vi "Diagnostics.Restart.Loop.vi"(8 "error in (no error)":errorcluster, 11 "State Variables Out":T1={"Comm"=refnum, "Parameters"={"Properties"={"Name"="", "CAN"={"Interface"="", "Baud Rate"=0, "Diagnostic Protocol"=enum."GMLAN", "Transport Protocol"=enum."ISO TP - Normal Mode", "Transmit ID"=0, "Receive ID"=0, "Transmit Extension"=2, "Receive Extension"=1, "Receive UUDT ID"=0, "Enable Stream"=TRUE, "VW TP Channel ID"=0, "Fill Frame"=FALSE, "Fill Byte"=255, "Termination"=FALSE, "LIN Cluster"="ADCS_LIN_database", "NAD"=1, "IO Mode"=0, "Max DLC"=8, "FD Baud Rate"=0, "Security"={"Source DLL Path"=path "", "Security Level"=0, "Target DLL Path"=path ""}}, "986x"={"Enable"=FALSE, "RIO Device"="", "Bitfile"=path ""}, "Reads"=[], "Frames Lookup"=variant(enum16{"GMLAN", "KWP-2000", "UDS"} enum."GMLAN"), "Writes"=[], "DPIDs"=[], "DPID Lookup"=variant(u32 0), "DTC"={"Descriptor"={"DTC Byte Length"=2, "Status Byte Length"=1, "Add Data Byte Length"=1, "Byte Order"=enum."Motorola"}, "Value.Code"=[], "Value.String"=[], "Value.J2012String"=[], "Status.Code"=[], "Status.String"=[]}, "Created DTCs"=0}}, "ADCS Connection"={"Diag CAN Handle"=0, "Transport Protocol"=enum."ISO TP - Normal Mode", "Receive Address Extension"=0, "Transmit Address Extension"=0, "Receive CAN Id"=0, "Transmit CAN Id"=0, "Log Frames ?"=FALSE, "My TP Address"=0, "Other TP Address"=0, "T1"=0, "T2"=0, "T3"=0, "T4"=0, "Tx SN"=0, "Block Size"=0, "Rx SN"=0, "VW TP Initialized?"=FALSE, "Tx block no"=0, "baud rate"=0, "Interface"="", "Channel Diag CAN Handle"=0, "UDP Connection ID"=refnum, "TCP Connection ID"=refnum, "Target IP Addr"=0, "Source Address"=0, "Target Address"=0, "Send Header NACK?"=FALSE, "DLL Handle"=0, "NAD"=0, "Time Stamp read first"=0.0, "Time Stamp read last"=0.0, "Time Stamp write first"=0.0, "Time Stamp write last"=0.0, "Time Stamp write"=0.0, "Time Stamp read"=0.0, " I/O Mode"=0, "FD Baudrate"=0, "TX_DL"=8, "RX_DL"=8, "DoIP Protocol Version"=1, " Selected I/O Mode"=0, "TesterPresent Counter"=0, "TesterPresent Limit"=0, "TesterPresent Tick[ms]"=10, "TesterPresent RequireResponse?"=FALSE, "TesterPresent Stored Ref?"=FALSE, "TesterPresent Message"=[], "TesterPresent Task Handle"=0, "TesterPresent Semaphore"=refnum, "Response Plausibility Check"=1, "Default Version?"=TRUE, "Diagostic Globals"={"Timeout FC (Bs)"=250, "Timeout CF (Cr)"=250, "Timeout Diag Command"=1000, "Receive Block Size (BS)"=0, "Wait Time CF (STmin)"=5, "Max Waits (N_WFTmax)"=10, "Waits to Send (N_WAIT)"=0, "Time between Waits (TW)"=25, "Fill CAN Frames?"=TRUE, "Fill Byte"=255, "Invalid Response as Error?"=FALSE, "Max RspPending Count"=5, "VWTP Command Timeout"=50, "Transport Protocol"=enum."Diagnostics on IP", "Diag CAN Handle"=0, "DLL Handle"=0, "Timeout RspPending"=1000}, "Session-based Properties?"=FALSE}, "XNET References"={"Database"="", "GMLAN DPID Session"="", "Cluster"=""}, "XNETEngine (GMLAN)"=refnum, "Process"=refnum, "Reads"=refnum, "Writes"=refnum, "Cmds"=refnum, "DTCs"=refnum, "DTC Count"=refnum, "Status"=refnum, "Triggers"=refnum, "CANConnected"=refnum, "LocalStop"=refnum, "LocalCommStatus"=refnum} {"ADCS Connection"."Diagostic Globals"."Fill Byte" format="%x"; "ADCS Connection"."TesterPresent Message" format="%.0x"; "ADCS Connection"."Selected I/O Mode" items=["CAN", "CAN FD", "CAN FD+BRS", "ECU Determined"]; "ADCS Connection"."DoIP Protocol Version" items=["2010"=1, "2012"=2]; "ADCS Connection"."RX_DL" items=["8"=8, "12"=12, "16"=16, "20"=20, "24"=24, "32"=32, "48"=48, "64"=64]; "ADCS Connection"."TX_DL" items=["8"=8, "12"=12, "16"=16, "20"=20, "24"=24, "32"=32, "48"=48, "64"=64]; "ADCS Connection"."I/O Mode" items=["CAN", "CAN FD", "CAN FD+BRS", "Not yet determined"]; "Parameters"."Properties"."Writes"."Signals"."Byte Order" items=["Little Endian", "Big Endian"]; "Parameters"."Properties"."Writes"."Signals"."Data Type" items=["Signed", "Unsigned", "IEEE Float"]; "Parameters"."Properties"."CAN"."IO Mode" items=["CAN 2.0", "CAN FD", "CAN FD+BRS"]; "Parameters"."Properties"."CAN"."Fill Byte" format="%.0x"; "Parameters"."Properties"."CAN"."VW TP Channel ID" format="%.0x"; "Parameters"."Properties"."CAN"."Receive UUDT ID" format="%.0x"; "Parameters"."Properties"."CAN"."Receive Extension" format="%.0x"; "Parameters"."Properties"."CAN"."Transmit Extension" format="%.0x"; "Parameters"."Properties"."CAN"."Receive ID" format="%.0x"; "Parameters"."Properties"."CAN"."Transmit ID" format="%.0x"; "Parameters"."Properties"."Reads"."Signals"."Byte Order" items=["Little Endian", "Big Endian"]; "Parameters"."Properties"."Reads"."Signals"."Data Type" items=["Signed", "Unsigned", "IEEE Float"]}) -> (0 "Error Out":errorcluster)   [LabVIEW 2019, in "Diagnostics Addon Engine.lvlib"]
uses:
  Diagnostics Addon Engine.lvlib
  Types/Diagnostics.State.ctl
  <vilib>/NI/NIVS Addon Network Comm/Engine/VeriStand Comm.lvclass
  <vilib>/NI/NIVS Inline Async API/_VS Inline Async API/Process/Process.lvclass
  Shared/Types/SysDef.Compile.ctl
  Shared/Types/SysDef.Compile.Properties.ctl
  Shared/Types/CAN.ctl
  Shared/Types/CAN.Interface.ctl
  Shared/Types/Protocol.ctl
  Shared/Types/Transport.ctl
  Shared/Types/Security.ctl
  Shared/Types/986x.ctl
  Shared/Types/Frame.Compile.ctl
  Shared/Types/Type.ctl
  Shared/Types/Signal.ctl
  Shared/Types/DPID.ctl
  Shared/Types/DPID.Rate.ctl
  Shared/Types/DTC.Settings.ctl
  Shared/Types/DTC.Descriptor.ctl
  <vilib>/Automotive Diagnostic Command Set/Diagnostic Transport.llb/Diag Reference.ctl
  <vilib>/Automotive Diagnostic Command Set/Diagnostic Transport.llb/Transport Protocol Selector.ctl
  <vilib>/Automotive Diagnostic Command Set/Diagnostic Transport.llb/DoIP Protocol Version.ctl
  <vilib>/Automotive Diagnostic Command Set/Diagnostic Transport.llb/Diag Globals.ctl
  Types/XNET.Refs.ctl
  <vilib>/NI/AMC/Message Queue.ctl
  <vilib>/NI/AMC/Message.ctl
  <vilib>/NI/Tools/Keyed Array/KeyedArray.ctl
  <vilib>/NI/NIVS Inline Async API/_Data Access Engine/Data Access Engine/Types/Write.DVR.ctl
  <vilib>/NI/NIVS Inline Async API/_Data Access Engine/Access Type Classes/Write/Write.lvclass
  <vilib>/NI/NIVS Inline Async API/_Data Access Engine/Data Access Engine/Types/Read.DVR.ctl
  <vilib>/NI/NIVS Inline Async API/_Data Access Engine/Access Type Classes/Read/Read.lvclass
  <vilib>/NI/NIVS Inline Async API/_Data Access Engine/Data Access Engine/Types/ReadWrite.DVR.ctl
  <vilib>/NI/NIVS Inline Async API/_Data Access Engine/Access Type Classes/ReadWrite/ReadWrite.lvclass
  <vilib>/NI/NIVS Inline Async API/_Data Access Engine/Access Type Classes/Write/Write.lvclass/Write.ctl
  <vilib>/NI/NIVS Addon Network Comm/Engine/VeriStand Comm.lvclass/VeriStand Comm.ctl
  <vilib>/NI/NIVS Inline Async API/_VS Inline Async API/Process/Process.lvclass/Process.ctl
  <vilib>/NI/NIVS Inline Async API/_Data Access Engine/Access Type Classes/Read/Read.lvclass/Read.ctl
  <vilib>/NI/NIVS Inline Async API/_Data Access Engine/Data Access Engine/Methods/Write.Data.vi
  Diagnostics.Main.UUDT.Engine.vi
  Diagnostics.Main.CmdResp.Engine.vi
  <vilib>/NI/NIVS Inline Async API/_VS Inline Async API/Error Handling Process/SubVIs/Error.ConvertArray.vi
  <vilib>/NI/NIVS Inline Async API/_Data Access Engine/Access Type Classes/Write/Write.ProcessData.vi
  <vilib>/NI/AMC/Read Next Message.vi
  <vilib>/NI/Tools/Keyed Array/Index.vi
  Frames.Refs.Cleanup.vi
  Status.Set.vi
  Signals.Scale.EU.vi
  <vilib>/NI/NIVS Inline Async API/_Data Access Engine/Data Access Engine/Methods/Write.Data.Commit.vi
  GMLAN/Utilities/Convert Data to DTCs.vi
  <vilib>/NI/NIVS Addon Network Comm/Engine/Comm API/Send Command.vi
  DTCs.List.Update.vi
  Restart.LocalStop.Read.vi
  GMLAN/_SubVIs/ReadDiagnosticInformation_ByStatus.vi
  GMLAN/_SubVIs/ReadDiagnosticInformation_sendOnChangeDTCCount.vi
  GMLAN/_SubVIs/ReadFailureRecordData_readFailureRecordParameters.vi
  GMLAN/_SubVIs/ReadDiagnosticInformation_readStatusOfDTCByDTCNumber.vi
  GMLAN/GMLAN DynamicallyDefineMessage.vi
  GMLAN/GMLAN ReadDataByPacketIdentifier.vi
  GMLAN/GMLAN ReadDataByParameterIdentifier.vi
  <vilib>/NI/AMC/Send Local Message.vi
  Signals.Scale.Raw.vi
  GMLAN/GMLAN DeviceControl.vi
  GMLAN/GMLAN TesterPresent.vi
  GMLAN/GMLAN InitiateDiagnosticOperation.vi
  GMLAN/GMLAN DisableNormalCommunication.vi
  GMLAN/GMLAN ReturnToNormalMode.vi
  ADCS.UnlockECUSecurity.vi
  <vilib>/NI/NIVS Addon Network Comm/Engine/Comm API/Respond to Command.vi
  DTC.Descriptor.Override.vi
  GMLAN/GMLAN ClearDiagnosticInformation.vi
  GMLAN/GMLAN ReadDataByIdentifier.vi
  Frames.Lookup.Size.Get.vi
  ADCS.TesterPresent.vi
  <vilib>/NI/AMC/Read Termination Message.vi
  <vilib>/NI/Tools/Keyed Array/Map String.vi
  ADCS.Get.ErrorByte.vi
  <vilib>/NI/NIVS Inline Async API/_Data Access Engine/Data Access Engine/Methods/Write.Data.Buffer.vi
  <vilib>/NI/NIVS Inline Async API/_Data Access Engine/Access Type Classes/Write/Write.Commit.vi
  GMLAN/Utilities/Convert Raw Data to DTCs.vi
  <vilib>/Utility/error.llb/Clear Errors.vi
  <vilib>/NI/AMC/Create Single Message.vi
  <vilib>/NI/AMC/Update Message Routing Info.vi
  <vilib>/NI/NIVS Inline Async API/_Data Access Engine/Data Access Engine/Methods/Read.Data.vi
  GMLAN/Utilities/GMLAN Service Broadcast.vi
  Security.DLL.vi
  GMLAN/GMLAN SecurityAccess.vi
  GMLAN/_SubVIs/SecurityAccess_sendKey.vi
  GMLAN/_SubVIs/SecurityAccess_requestSeed.vi
  <vilib>/NI/Tools/String/Get Case Matching.vi
  <vilib>/NI/NIVS Inline Async API/_Data Access Engine/Access Type Classes/Write/Write.Buffer.vi
  <vilib>/NI/NIVS Inline Async API/_Data Access Engine/Access Type Classes/Read/Read.ProcessData.vi
  <vilib>/Automotive Diagnostic Command Set/Diagnostic Transport.llb/Diagnostic Service Send.vi
  <vilib>/Automotive Diagnostic Command Set/Diagnostic Transport.llb/Diagnostic Response Recv.vi
  <vilib>/Automotive Diagnostic Command Set/Diagnostic Transport.llb/ISOTP Transmit.vi
  <vilib>/Automotive Diagnostic Command Set/Diagnostic Transport.llb/ISOTP7 Transmit.vi
  <vilib>/Automotive Diagnostic Command Set/Diagnostic Transport.llb/DoIP Transmit.vi
  <vilib>/Automotive Diagnostic Command Set/Diagnostic Transport.llb/LIN ISOTP Transmit.vi
  <vilib>/Automotive Diagnostic Command Set/Diagnostic Transport.llb/Diagnostic Service Recv.vi
  <vilib>/Automotive Diagnostic Command Set/Diagnostic Transport.llb/ISOTP Send FF.vi
  <vilib>/Automotive Diagnostic Command Set/Diagnostic Transport.llb/ISOTP Send CFs.vi
  <vilib>/Automotive Diagnostic Command Set/Diagnostic Transport.llb/ISOTP Send Frame.vi
  <vilib>/Automotive Diagnostic Command Set/Diagnostic Transport.llb/ISOTP7 Send FF.vi
  <vilib>/Automotive Diagnostic Command Set/Diagnostic Transport.llb/ISOTP7 Send CFs.vi
  <vilib>/Automotive Diagnostic Command Set/Diagnostic Transport.llb/ISOTP7 Send Frame.vi
  <vilib>/Automotive Diagnostic Command Set/Diagnostic Transport.llb/DoIP TCP Msg Send.vi
  <vilib>/Automotive Diagnostic Command Set/Diagnostic Transport.llb/DoIP TCP Msg Recv.vi
  <vilib>/Automotive Diagnostic Command Set/Diagnostic Transport.llb/DoIP Check Addresses.vi
  <vilib>/Automotive Diagnostic Command Set/Diagnostic Transport.llb/DoIP Check ACK Code.vi
  <vilib>/Automotive Diagnostic Command Set/Diagnostic Transport.llb/ISOTP Receive.vi
  <vilib>/Automotive Diagnostic Command Set/Diagnostic Transport.llb/ISOTP7 Receive.vi
  <vilib>/Automotive Diagnostic Command Set/Diagnostic Transport.llb/DoIP Receive.vi
  <vilib>/Automotive Diagnostic Command Set/Diagnostic Transport.llb/LIN ISOTP Receive.vi
  <vilib>/Automotive Diagnostic Command Set/Diagnostic Transport.llb/Diag Get Globals.vi
  <vilib>/Automotive Diagnostic Command Set/Diagnostic Transport.llb/ISOTP Recv FC.vi
  <vilib>/Automotive Diagnostic Command Set/Diagnostic Transport.llb/ISOTP Send CF.vi
  <vilib>/Automotive Diagnostic Command Set/Diagnostic Transport.llb/Diag Fill Frame.vi
  <vilib>/Automotive Diagnostic Command Set/Diagnostic Transport.llb/ISOTP Calc Send Params.vi
  <vilib>/Automotive Diagnostic Command Set/Diagnostic Transport.llb/ISOTP7 Recv FC.vi
  <vilib>/Automotive Diagnostic Command Set/Diagnostic Transport.llb/ISOTP7 Send CF.vi
  <vilib>/Automotive Diagnostic Command Set/Diagnostic Transport.llb/DoIP Add Addresses.vi
  <vilib>/Automotive Diagnostic Command Set/Diagnostic Transport.llb/DoIP TCP Send.vi
  <vilib>/Automotive Diagnostic Command Set/Diagnostic Transport.llb/DoIP TCP Recv.vi
  <vilib>/Automotive Diagnostic Command Set/Diagnostic Transport.llb/DoIP Add Header.vi
  <vilib>/Automotive Diagnostic Command Set/Diagnostic Transport.llb/ISOTP Recv Frame.vi
  <vilib>/Automotive Diagnostic Command Set/Diagnostic Transport.llb/ISOTP Recv CFs.vi
  <vilib>/Automotive Diagnostic Command Set/Diagnostic Transport.llb/ISOTP7 Recv Frame.vi
  <vilib>/Automotive Diagnostic Command Set/Diagnostic Transport.llb/ISOTP7 Recv CFs.vi
  <vilib>/Automotive Diagnostic Command Set/Diagnostic Transport.llb/DoIP Send Alive.vi
  <vilib>/Automotive Diagnostic Command Set/Diagnostic Transport.llb/DoIP Check Error.vi
  <vilib>/Automotive Diagnostic Command Set/Diagnostic Transport.llb/ISOTP Check Redo.vi
  <vilib>/Automotive Diagnostic Command Set/Diagnostic Transport.llb/ISOTP Recv Block.vi
  <vilib>/Automotive Diagnostic Command Set/Diagnostic Transport.llb/ISOTP7 Recv Block.vi
  <vilib>/Automotive Diagnostic Command Set/Diagnostic Transport.llb/ISOTP Send FC.vi
  <vilib>/Automotive Diagnostic Command Set/Diagnostic Transport.llb/ISOTP Add CF.vi
  <vilib>/Automotive Diagnostic Command Set/Diagnostic Transport.llb/ISOTP7 Send FC.vi
  <vilib>/Automotive Diagnostic Command Set/Diagnostic Transport.llb/ISOTP7 Add CF.vi
  <vilib>/NI/NIVS Addon Network Comm/Shared/Comm Constants.vi
  <vilib>/NI/AMC/Globals.vi
  <vilib>/Automotive Diagnostic Command Set/Diagnostic Transport.llb/Diag Get Property.vi
  <vilib>/Automotive Diagnostic Command Set/Diagnostic Transport.llb/Diag Set Property.vi
  <vilib>/Automotive Diagnostic Command Set/Diagnostic Transport.llb/Diagnostic Service.vi
  <vilib>/Automotive Diagnostic Command Set/Diagnostic Transport.llb/Apply Success Failure Error.vi
  DPIDs.IDs.Sort.vi
  <vilib>/NI/AMC/Send Message.vi
  Shared/SubVIs/Constants.vi
  <vilib>/xnet/xnet.llb/XNET Convert.vi
  <vilib>/xnet/xnet.llb/XNET Convert (Signal to Frame CAN).vi
  <vilib>/Automotive Diagnostic Command Set/Diagnostic Protocols.llb/TesterPresent.vi
  <vilib>/Automotive Diagnostic Command Set/Diagnostic Transport.llb/Diag Globals.vi
  <vilib>/Automotive Diagnostic Command Set/Diagnostic Transport.llb/CAN Send Frame Check Queue.vi
  <vilib>/Automotive Diagnostic Command Set/Diagnostic Transport.llb/Diag CAN get timestamp.vi
  <vilib>/Automotive Diagnostic Command Set/Diagnostic Transport.llb/Diag CAN read.vi
  <vilib>/Automotive Diagnostic Command Set/Diagnostic Transport.llb/ISOTP Calc Actual IO Mode.vi
  <vilib>/Automotive Diagnostic Command Set/Diagnostic Transport.llb/ISOTP Get FC Data.vi
  <vilib>/Automotive Diagnostic Command Set/Diagnostic Transport.llb/VWTP Write.vi
  <vilib>/Automotive Diagnostic Command Set/Diagnostic Transport.llb/DoIP Analyze Header.vi
  <vilib>/Automotive Diagnostic Command Set/Diagnostic Transport.llb/Diag CAN status.vi
  <vilib>/Automotive Diagnostic Command Set/Diagnostic Transport.llb/VWTP Read.vi
  <vilib>/Automotive Diagnostic Command Set/Diagnostic Transport.llb/Apply Diagnostic Error.vi
  <vilib>/Automotive Diagnostic Command Set/Diagnostic Protocols.llb/UDS TesterPresent.vi
  <vilib>/Automotive Diagnostic Command Set/Diagnostic Protocols.llb/UDS DiagnosticSessionControl.vi
  <vilib>/Automotive Diagnostic Command Set/Diagnostic Protocols.llb/StartDiagnosticSession.vi
  <vilib>/Automotive Diagnostic Command Set/Diagnostic Protocols.llb/StopDiagnosticSession.vi
  <vilib>/Automotive Diagnostic Command Set/Diagnostic Protocols.llb/UDS CommunicationControl.vi
  <vilib>/Automotive Diagnostic Command Set/Diagnostic Protocols.llb/DisableNormalMessageTransmission.vi
  <vilib>/Automotive Diagnostic Command Set/Diagnostic Protocols.llb/EnableNormalMessageTransmission.vi
  <vilib>/Automotive Diagnostic Command Set/Diagnostic Protocols.llb/UDS RequestSeed.vi
  <vilib>/Automotive Diagnostic Command Set/Diagnostic Protocols.llb/RequestSeed.vi
  <vilib>/Automotive Diagnostic Command Set/Diagnostic Protocols.llb/UDS SendKey.vi
  <vilib>/Automotive Diagnostic Command Set/Diagnostic Protocols.llb/SendKey.vi
  <vilib>/Automotive Diagnostic Command Set/Diagnostic Protocols.llb/UDS ReportDTCBySeverityMaskRecord.vi
  <vilib>/Automotive Diagnostic Command Set/Diagnostic Protocols.llb/UDS ReportSeverityInformationOfDTC.vi
  <vilib>/Automotive Diagnostic Command Set/Diagnostic Protocols.llb/UDS ReportDTCByStatusMask.vi
  <vilib>/Automotive Diagnostic Command Set/Diagnostic Protocols.llb/ReadStatusOfDTC.vi
  <vilib>/Automotive Diagnostic Command Set/Diagnostic Protocols.llb/ReadDTCByStatus.vi
  <vilib>/Automotive Diagnostic Command Set/Diagnostic Protocols.llb/ClearDiagnosticInformation.vi
  <vilib>/Automotive Diagnostic Command Set/Diagnostic Protocols.llb/UDS ClearDiagnosticInformation.vi
  <vilib>/Automotive Diagnostic Command Set/Diagnostic Protocols.llb/ReadDataByLocalIdentifier.vi
  <vilib>/Automotive Diagnostic Command Set/Diagnostic Protocols.llb/UDS ReadDataByIdentifier.vi
  <vilib>/xnet/xnet.llb/XNET Convert (Frame CAN to Signal).vi
  <vilib>/Automotive Diagnostic Command Set/Diagnostic Protocols.llb/WriteDataByLocalIdentifier.vi
  <vilib>/Automotive Diagnostic Command Set/Diagnostic Protocols.llb/UDS WriteDataByIdentifier.vi
  <vilib>/Automotive Diagnostic Command Set/Diagnostic Protocols.llb/UDS ControlDTCSetting.vi
  <vilib>/Automotive Diagnostic Command Set/Diagnostic Protocols.llb/ControlDTCSetting.vi
  <vilib>/Automotive Diagnostic Command Set/Diagnostic Protocols.llb/ECUReset.vi
  <vilib>/Automotive Diagnostic Command Set/Diagnostic Protocols.llb/UDS ECUReset.vi
  <vilib>/Automotive Diagnostic Command Set/Diagnostic Protocols.llb/ReadMemoryByAddress.vi
  <vilib>/Automotive Diagnostic Command Set/Diagnostic Protocols.llb/UDS06 ReadMemoryByAddress.vi
  <vilib>/Automotive Diagnostic Command Set/Diagnostic Protocols.llb/UDS ReadMemoryByAddress.vi
  <vilib>/Automotive Diagnostic Command Set/Diagnostic Protocols.llb/WriteMemoryByAddress.vi
  <vilib>/Automotive Diagnostic Command Set/Diagnostic Protocols.llb/UDS06 WriteMemoryByAddress.vi
  <vilib>/Automotive Diagnostic Command Set/Diagnostic Protocols.llb/UDS WriteMemoryByAddress.vi
  <vilib>/Automotive Diagnostic Command Set/Diagnostic Protocols.llb/InputOutputControlByLocalIdentifier.vi
  <vilib>/Automotive Diagnostic Command Set/Diagnostic Protocols.llb/UDS InputOutputControlByIdentifier.vi
  <vilib>/Automotive Diagnostic Command Set/Diagnostic Protocols.llb/StartRoutineByLocalIdentifier.vi
  <vilib>/Automotive Diagnostic Command Set/Diagnostic Protocols.llb/UDS RoutineControl.vi
  <vilib>/Automotive Diagnostic Command Set/Diagnostic Protocols.llb/RequestRoutineResultsByLocalIdentifier.vi
  <vilib>/Automotive Diagnostic Command Set/Diagnostic Protocols.llb/StopRoutineByLocalIdentifier.vi
  <vilib>/xnet/xnet.llb/XNET Read.vi
  <vilib>/xnet/xnet.llb/XNET Read (Frame CAN).vi
  <vilib>/Automotive Diagnostic Command Set/Diagnostic Protocols.llb/Convert to Phys.vi
  <vilib>/xnet/xnet.llb/XNET Clear.vi
  <vilib>/xnet/xnet.llb/XNET Database Delete Object.vi
  <vilib>/xnet/xnet.llb/XNET Database Delete (Cluster).vi
  <vilib>/xnet/xnet.llb/XNET Database Close.vi
  <vilib>/xnet/xnet.llb/XNET Database Close (Database).vi
  <vilib>/Automotive Diagnostic Command Set/Diagnostic Transport.llb/Close Diagnostic.vi
  <vilib>/NI VeriStand/Custom Device Tools/Custom Device Utility Library/Custom Device Utility Library.lvlib
  <vilib>/NI/NIVS Inline Async API/_Data Access Engine/Data Access Engine/Data Access Engine.lvclass
  Shared/Diagnostics Addon Shared.lvlib
  <vilib>/addons/Automotive Diagnostic Command Set/NI_Automotive Diagnostic Command Set.lvlib
  <vilib>/NI/Tools/Keyed Array/Tools_KeyedArray.lvlib
  <vilib>/NI/AMC/AMC.lvlib
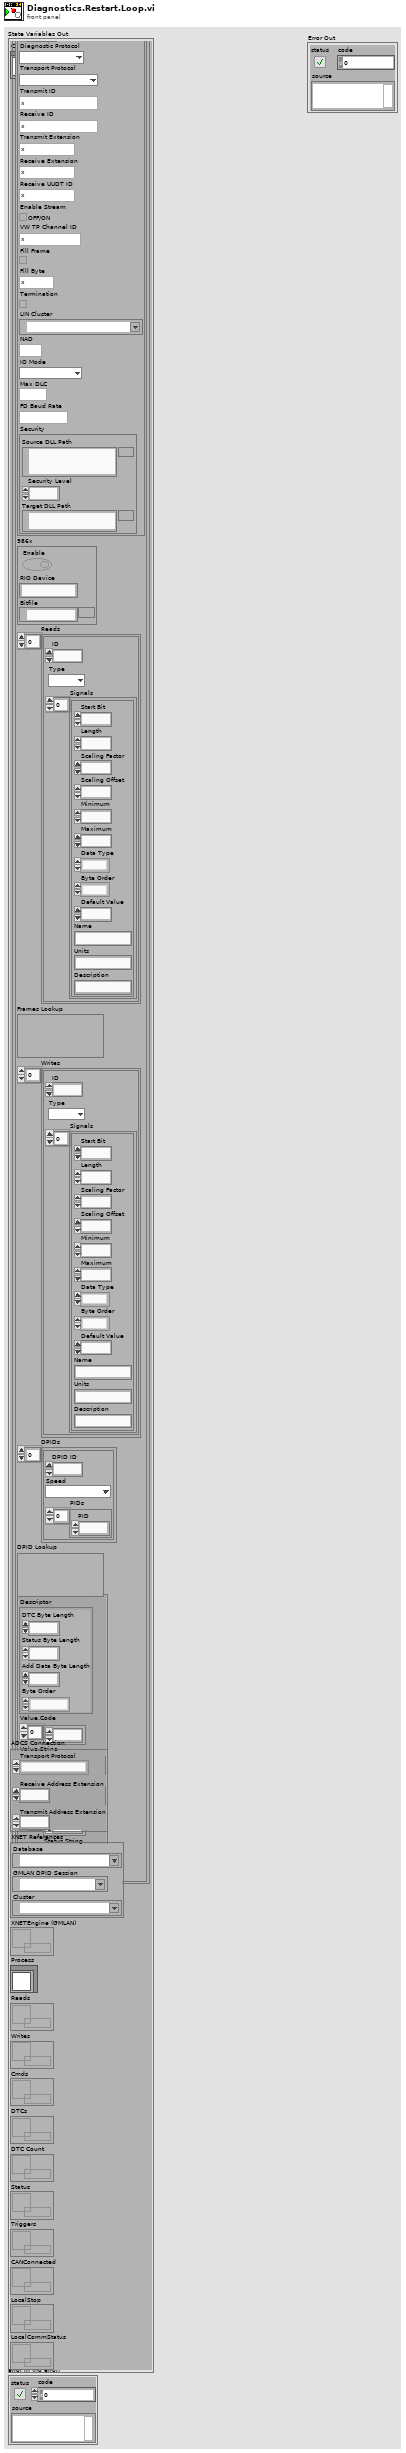
[diagram p1: front panel]
types:
  T1 = typedef "Diagnostics Addon Engine.lvlib/Diagnostics.State.ctl" = cluster{"Comm":refnum<class "VeriStand Comm.lvclass">, "Parameters":T2, "ADCS Connection":T17, "XNET References":T22, "XNETEngine (GMLAN)":T23, "Process":refnum<class "Process.lvclass">, "Reads":T24, "Writes":T25, "Cmds":T26, "DTCs":T24, "DTC Count":T24, "Status":T24, "Triggers":T26, "CANConnected":T24, "LocalStop":refnum<data-value>, "LocalCommStatus":refnum<data-value>}
  T2 = typedef "Diagnostics Addon Shared.lvlib/SysDef.Compile.ctl" = cluster{"Properties":T3}
  T3 = typedef "Diagnostics Addon Shared.lvlib/SysDef.Compile.Properties.ctl" = cluster{"Name":string, "CAN":T4, "986x":T9, "Reads":T10[], "Frames Lookup":variant, "Writes":T10[], "DPIDs":T13[], "DPID Lookup":variant, "DTC":T15, "Created DTCs":u32}
  T4 = typedef "Diagnostics Addon Shared.lvlib/CAN.ctl" = cluster{"Interface":T5, "Baud Rate":u64, "Diagnostic Protocol":T6, "Transport Protocol":T7, "Transmit ID":u32, "Receive ID":u32, "Transmit Extension":u8, "Receive Extension":u8, "Receive UUDT ID":u32, "Enable Stream":bool, "VW TP Channel ID":u32, "Fill Frame":bool, "Fill Byte":u8, "Termination":bool, "LIN Cluster":refnum<k21>, "NAD":u8, "IO Mode":u32, "Max DLC":u16, "FD Baud Rate":u64, "Security":T8}
  T5 = typedef "Diagnostics Addon Shared.lvlib/CAN.Interface.ctl" = string
  T6 = typedef "Diagnostics Addon Shared.lvlib/Protocol.ctl" = enum16{"GMLAN", "KWP-2000", "UDS", "User-Defined"}
  T7 = typedef "Diagnostics Addon Shared.lvlib/Transport.ctl" = enum16{"ISO TP - Normal Mode", "ISO TP - Mixed Mode", "VW TP 2.0", "Diagnostics on IP", "ISO TP LIN"}
  T8 = typedef "Diagnostics Addon Shared.lvlib/Security.ctl" = cluster{"Source DLL Path":path, "Security Level":u8, "Target DLL Path":path}
  T9 = typedef "Diagnostics Addon Shared.lvlib/986x.ctl" = cluster{"Enable":bool, "RIO Device":string, "Bitfile":path}
  T10 = typedef "Diagnostics Addon Shared.lvlib/Frame.Compile.ctl" = cluster{"ID":u32, "Type":T11, "Signals":T12[]}
  T11 = typedef "Diagnostics Addon Shared.lvlib/Type.ctl" = enum16{"DID", "CDID", "PID", "CPID", "Read Memory", "Write Memory", "DTC Control", "IO Cmd", "IO Resp", "Routine Start Cmd", "Routine Start Resp", "Routine Request Cmd", "Routine Request Resp", "Routine Stop Cmd", "Routine Stop Resp", "UserDefined Cmd", "UserDefined Rsp"}
  T12 = typedef "Diagnostics Addon Shared.lvlib/Signal.ctl" = cluster{"Start Bit":u32, "Length":u32, "Scaling Factor":dbl, "Scaling Offset":dbl, "Minimum":dbl, "Maximum":dbl, "Data Type":u32, "Byte Order":u32, "Default Value":dbl, "Name":string, "Units":string, "Description":string}
  T13 = typedef "Diagnostics Addon Shared.lvlib/DPID.ctl" = cluster{"DPID ID":u8, "Speed":T14, "PIDs":u16[]}
  T14 = typedef "Diagnostics Addon Shared.lvlib/DPID.Rate.ctl" = enum16{"Slow", "Medium", "Fast"}
  T15 = typedef "Diagnostics Addon Shared.lvlib/DTC.Settings.ctl" = cluster{"Descriptor":T16, "Value.Code":dbl[], "Value.String":string[], "Value.J2012String":string[], "Status.Code":dbl[], "Status.String":string[]}
  T16 = typedef "Diagnostics Addon Shared.lvlib/DTC.Descriptor.ctl" = cluster{"DTC Byte Length":i32, "Status Byte Length":i32, "Add Data Byte Length":i32, "Byte Order":enum16{"Motorola", "Intel"}}
  T17 = typedef "NI_Automotive Diagnostic Command Set.lvlib/Diag Reference.ctl" = cluster{"Diag CAN Handle":u32, "Transport Protocol":T18, "Receive Address Extension":u8, "Transmit Address Extension":u8, "Receive CAN Id":u32, "Transmit CAN Id":u32, "Log Frames ?":bool, "My TP Address":u8, "Other TP Address":u8, "T1":u16, "T2":u16, "T3":u16, "T4":u16, "Tx SN":u8, "Block Size":u8, "Rx SN":u8, "VW TP Initialized?":bool, "Tx block no":u8, "baud rate":u64, "Interface":string, "Channel Diag CAN Handle":u32, "UDP Connection ID":refnum<k16>, "TCP Connection ID":refnum<k5>, "Target IP Addr":u32, "Source Address":u16, "Target Address":u16, "Send Header NACK?":bool, "DLL Handle":u32, "NAD":u8, "Time Stamp read first":dbl, "Time Stamp read last":dbl, "Time Stamp write first":dbl, "Time Stamp write last":dbl, "Time Stamp write":dbl, "Time Stamp read":dbl, " I/O Mode":u32, "FD Baudrate":u64, "TX_DL":u16, "RX_DL":u16, "DoIP Protocol Version":T19, " Selected I/O Mode":u32, "TesterPresent Counter":u32, "TesterPresent Limit":u32, "TesterPresent Tick[ms]":i32, "TesterPresent RequireResponse?":bool, "TesterPresent Stored Ref?":bool, "TesterPresent Message":u8[], "TesterPresent Task Handle":i32, "TesterPresent Semaphore":T20, "Response Plausibility Check":u32, "Default Version?":bool, "Diagostic Globals":T21, "Session-based Properties?":bool}
  T18 = typedef "NI_Automotive Diagnostic Command Set.lvlib/Transport Protocol Selector.ctl" = enum16{"ISO TP - Normal Mode", "ISO TP - Mixed Mode", "VW TP 2.0", "Diagnostics on IP", "ISO TP LIN"}
  T19 = typedef "NI_Automotive Diagnostic Command Set.lvlib/DoIP Protocol Version.ctl" = u8
  T20 = typedef "Semaphore RefNum" = refnum<k1>
  T21 = typedef "NI_Automotive Diagnostic Command Set.lvlib/Diag Globals.ctl" = cluster{"Timeout FC (Bs)":u32, "Timeout CF (Cr)":u32, "Timeout Diag Command":u32, "Receive Block Size (BS)":u8, "Wait Time CF (STmin)":u8, "Max Waits (N_WFTmax)":u8, "Waits to Send (N_WAIT)":i32, "Time between Waits (TW)":u32, "Fill CAN Frames?":bool, "Fill Byte":u32, "Invalid Response as Error?":bool, "Max RspPending Count":u32, "VWTP Command Timeout":u32, "Transport Protocol":T18, "Diag CAN Handle":u32, "DLL Handle":u32, "Timeout RspPending":u32}
  T22 = typedef "Diagnostics Addon Engine.lvlib/XNET.Refs.ctl" = cluster{"Database":refnum<k21>, "GMLAN DPID Session":refnum<k21>, "Cluster":refnum<k21>}
  T23 = typedef "AMC.lvlib/Message Queue.ctl" = refnum<queue>
  T24 = typedef "Data Access Engine.lvlib/Data Access Engine.lvclass/Write.DVR.ctl" = refnum<data-value>
  T25 = typedef "Data Access Engine.lvlib/Data Access Engine.lvclass/Read.DVR.ctl" = refnum<data-value>
  T26 = typedef "Data Access Engine.lvlib/Data Access Engine.lvclass/ReadWrite.DVR.ctl" = refnum<data-value>
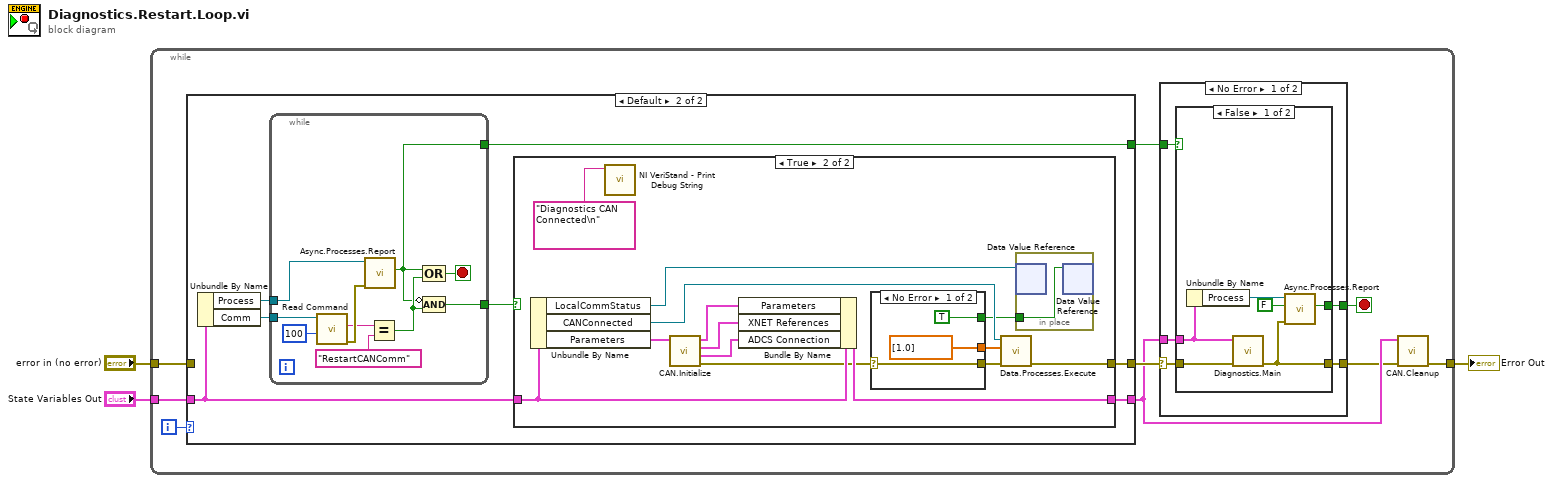
[diagram p0: block diagram]
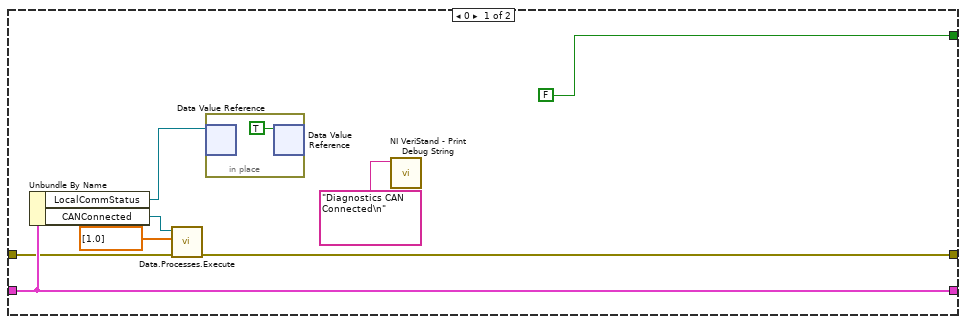
[diagram p2: hidden frame]
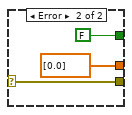
[diagram p4: hidden frame]
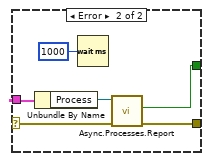
[diagram p6: hidden frame]
diagram:
  n1 = while {
    tunnel: "error in (no error)" -> [w12]
    tunnel: "State Variables Out" -> [w11]
    tunnel: [w5] -> w1
    i -> [w8]
    stop <- w9 stop-if-true
    n2 = case shown="Default" w8 {
      tunnel: [w20 w28] -> w7
      tunnel: w12 -> [w18 _]
      tunnel: w11 -> [w20 w26]
      tunnel: [w17 w27] -> w10
      tunnel: [FALSE w22] -> w4
      frame 0 {
        n3 = Unbundle By Name(w20) -> ("LocalCommStatus"=w13:refnum<data-value>, "CANConnected"=w19:T24)
        n4 = call-poly <vilib>:"Data.Processes.Execute.vi"("error in (no error)"=w18, "Values"=dbl[] [1.0], "Ref"=w19) -> ("error out"=w17:errorcluster)  [unwired: 8 in]
        n5 = in-place {
          n6 = in-place-dvr #1(w13) -> ()  [unwired: 2 out]
          n7 = in-place-dvr #1(TRUE ("data value")) -> ()  [unwired: 2 out]
        }
        n8 = call <vilib>:"NI VeriStand - Print Debug String.vi"("Message"="Diagnostics CAN Connected\n") -> ()  [unwired: 10 in, 1 out]
      }
      frame Default {
        n9 = Unbundle By Name(w26) -> ("Process"=w24:refnum<class "Process.lvclass">, "Comm"=w25:refnum<class "VeriStand Comm.lvclass">)
        n10 = while {
          tunnel: w25 -> [w59]
          tunnel: w24 -> [w58]
          tunnel: [w52] -> w23
          tunnel: [w51] -> w22
          stop <- w54 stop-if-true
          n11 = call <vilib>:"Read Command.vi"("timeout (100 ms)"=100 ("timeout (1ms)"), "VeriStand Comm in"=w59) -> ("error out"=w57:errorcluster, "message name"=w55:string)  [unwired: 4 in, 4 out]
          n12 = call <vilib>:"Async.Processes.Report.vi"("Error"=w57, "Process in"=w58) -> ("Stop"=w51:bool)  [unwired: 8 in, 1 out]
          n13 = Equal?(x=w55, y="RestartCANComm" ("Name")) -> (x = y?=w53:bool)
          n14 = Compound Arithmetic op=OR(w51, w53) -> (w54:bool)
          n15 = Compound Arithmetic op=AND(invert w51, w53) -> (w52:bool)
        }
        n16 = case shown="True" w23 {
          tunnel: [w29 w43] -> w28
          tunnel: [_ w37] -> w27
          tunnel: w26 -> [w29 w35]
          frame False {
          }
          frame True {
            n17 = Unbundle By Name(w35) -> ("LocalCommStatus"=w33:refnum<data-value>, "CANConnected"=w36:T24, "Parameters"=w42:T2)
            n18 = call <vilib>:"NI VeriStand - Print Debug String.vi"("Message"="Diagnostics CAN Connected\n") -> ()  [unwired: 10 in, 1 out]
            n19 = call "CAN.Initialize.vi"("Parameters"=w42) -> ("error out"=w32:errorcluster, "ADCS Connection"=w39:T17, "XNET References"=w40:T22, "Parameters"=w41:T2)  [unwired: 7 in]
            n20 = Bundle By Name(cluster=w35, "Parameters"=w41, "XNET References"=w40, "ADCS Connection"=w39) -> (w43:T1)
            n21 = case shown="No Error" w32 {
              selector: w32 -> [w45 w49]
              tunnel: [dbl[] [1.0] ("Values") dbl[] [0.0] ("Values")] -> w38
              tunnel: [w45 w49] -> w31
              tunnel: [TRUE FALSE] -> w30
              frame No Error {
              }
              frame Error {
              }
            }
            n22 = call-poly <vilib>:"Data.Processes.Execute.vi"("error in (no error)"=w31, "Values"=w38, "Ref"=w36) -> ("error out"=w37:errorcluster)  [unwired: 8 in]
            n23 = in-place {
              in-place-border: w30 -> [w50]
              n24 = in-place-dvr #2(w33) -> ()  [unwired: 2 out]
              n25 = in-place-dvr #2(w50) -> ()  [unwired: 2 out]
            }
          }
        }
      }
    }
    n26 = case shown="No Error" w10 {
      selector: w10 -> [w63 w75]
      tunnel: w7 -> [w65 w78]
      tunnel: [w64 w74] -> w9
      tunnel: [w62 w75] -> w6
      tunnel: w4 -> [w61 _]
      frame No Error {
        n27 = case shown="False" w61 {
          selector: w61 -> [_ w72]
          tunnel: w65 -> [w71 _]
          tunnel: [w70 w72] -> w64
          tunnel: w63 -> [w69 w73]
          tunnel: [w68 w73] -> w62
          frame False {
            n28 = Unbundle By Name(w71) -> ("Process"=w67:refnum<class "Process.lvclass">)
            n29 = call "Diagnostics.Main.vi"("error in (no error)"=w69, "State Variables"=w71) -> ("error out"=w68:errorcluster)  [unwired: 9 in]
            n30 = call <vilib>:"Async.Processes.Report.vi"("Error"=w68, "Stop Async on Error?"=FALSE ("Stop on Error?"), "Process in"=w67) -> ("Stop"=w70:bool)  [unwired: 7 in, 1 out]
          }
          frame True {
          }
        }
      }
      frame Error {
        n31 = Unbundle By Name(w78) -> ("Process"=w77:refnum<class "Process.lvclass">)
        n32 = Wait (ms)(milliseconds to wait=u32 1000 ("millisecond multiple")) -> ()  [unwired: 1 out]
        n33 = call <vilib>:"Async.Processes.Report.vi"("Error"=w75, "Process in"=w77) -> ("Stop"=w74:bool)  [unwired: 8 in, 1 out]
      }
    }
    n34 = call "CAN.Cleanup.vi"("error in (no error)"=w6, "State Variables Out"=w7) -> ("error out"=w5:errorcluster)  [unwired: 9 in]
  }
  "Error Out" <- w1
